vi "Carriage Intake Test.vi"   [LabVIEW 2018]
uses:
  Floating Intake/Implementation/Floating Intake Operations.ctl
  <vilib>/Rock Robotics/Network Tables/NT Write String.vi
types:
  T1 = typedef "Floating Intake Operations.ctl" = enum16{"Reserve", "Read Current", "Immediate"}
  T2 = typedef "Command Status Info.ctl" = cluster{"Name":string, "Status":T3, "notifier out":T4}
  T3 = typedef "Completion Status.ctl" = enum16{"Successful", "Aborted", "Incomplete"}
  T4 = typedef "Completion Notifier.ctl" = refnum<notifier>
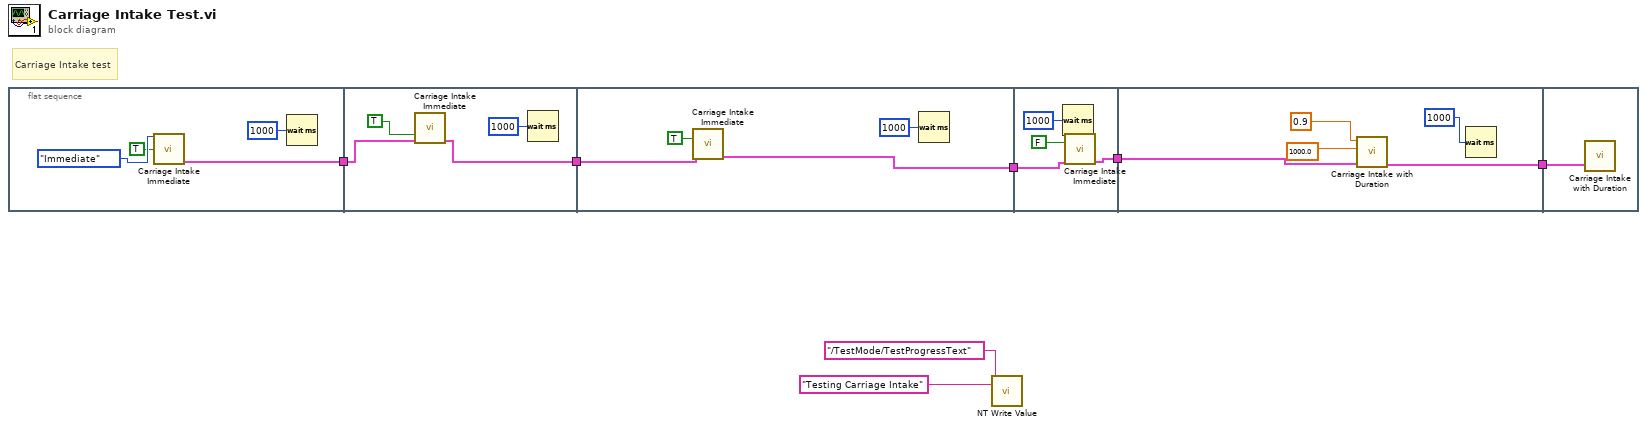
[diagram p0: block diagram]
diagram:
  # "Carriage Intake test"
  n1 = flat-sequence {
    tunnel: [w10] -> w7
    tunnel: w7 -> [w15]
    tunnel: [w14] -> w6
    tunnel: w6 -> [w19]
    tunnel: [w17] -> w5
    tunnel: w5 -> [w23]
    tunnel: [w22] -> w4
    tunnel: w4 -> [w26]
    tunnel: [w25] -> w3
    tunnel: w3 -> [w29]
    frame #0 {
      n2 = call "Carriage Intake Immediate.vi"("Setpoint"=Floating_Intake_Operations."Immediate" ("Operation"), "Open"=TRUE) -> ("Command Info Out"=w10:T2)  [unwired: 13 in]
      n3 = Wait (ms)(milliseconds to wait=u32 1000) -> ()  [unwired: 1 out]
    }
    frame #1 {
      n4 = call "Carriage Intake Immediate.vi"("Close"=TRUE, "Command Info In"=w15) -> ("Command Info Out"=w14:T2)  [unwired: 13 in]
      n5 = Wait (ms)(milliseconds to wait=u32 1000) -> ()  [unwired: 1 out]
    }
    frame #2 {
      n6 = call "Carriage Intake Immediate.vi"("Extend"=TRUE, "Command Info In"=w19) -> ("Command Info Out"=w17:T2)  [unwired: 13 in]
      n7 = Wait (ms)(milliseconds to wait=u32 1000) -> ()  [unwired: 1 out]
    }
    frame #3 {
      n8 = Wait (ms)(milliseconds to wait=u32 1000) -> ()  [unwired: 1 out]
      n9 = call "Carriage Intake Immediate.vi"("Extend"=FALSE, "Command Info In"=w23) -> ("Command Info Out"=w22:T2)  [unwired: 13 in]
    }
    frame #4 {
      n10 = call "Carriage Intake with Duration.vi"("Command Info In"=w26, "Duration (s)"=1000.0, "Setpoint"=0.9) -> ("Command Info Out"=w25:T2)  [unwired: 8 in]
      n11 = Wait (ms)(milliseconds to wait=u32 1000) -> ()  [unwired: 1 out]
    }
    frame #5 {
      n12 = call "Carriage Intake with Duration.vi"("Command Info In"=w29) -> ()  [unwired: 10 in, 1 out]
    }
  }
  n13 = call-poly <vilib>:"NT Write Value.vi"("String"="Testing Carriage Intake", "Name"="/TestMode/TestProgressText") -> ()  [unwired: 9 in, 1 out]
